vi "Boolean click counter program.vi"() -> ()   [LabVIEW 2021]
panel:
  out "Counts OFF":bool
  out "Turned off":dbl
  in  "Stop While":bool
  out "Turned on":dbl
  in  "Counts ON":bool
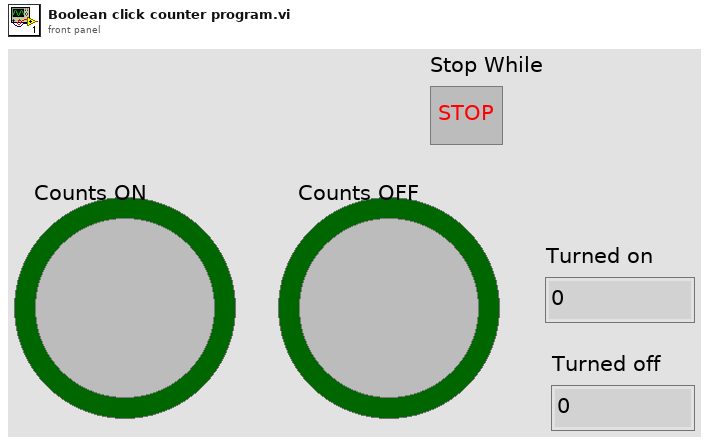
[diagram p1: front panel]
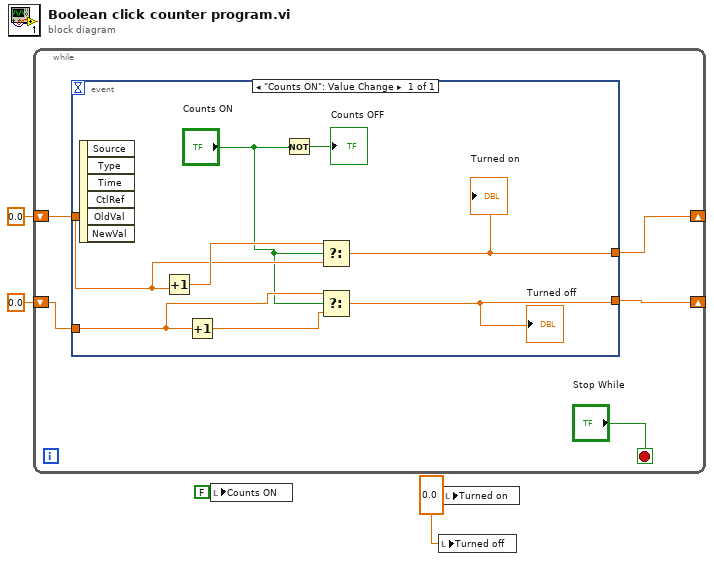
[diagram p0: block diagram]
diagram:
  w3 = 0.0 ("Numeric")
  n1 = while {
    shift-right: [w8] -> _
    shift-left: 0.0 -> [w9]
    shift-right: [w5] -> _
    shift-left: 0.0 -> [w6]
    stop <- "Stop While" stop-if-true
    n2 = event shown="[0] \"Counts ON\": Value Change" {
      selector: _ -> [_]
      dyn-events: _ -> [_]
      timeout: _ -> [_]
      tunnel: w9 -> [w15]
      tunnel: [w16] -> w8
      tunnel: w6 -> [w13]
      tunnel: [w12] -> w5
      event "Counts ON": Value Change {
        n3 = event-data() -> ()  [unwired: 1 in, 6 out]
        n4 = Increment(x=w15) -> (x+1=w17:dbl)
        n5 = Increment(x=w13) -> (x+1=w14:dbl)
        n6 = Not(x="Counts ON") -> (.not. x?=→"Counts OFF":bool)
        n7 = Select(t=w17, s="Counts ON", f=w15) -> (s? t:f=w16:dbl)
        "Turned on" <- w16
        n8 = Select(t=w13, s="Counts ON", f=w14) -> (s? t:f=w12:dbl)
        "Turned off" <- w12
      }
    }
  }
  n9 = local write "Counts ON"(FALSE ("Boolean")) -> ()
  n10 = local write "Turned off"(w3) -> ()
  n11 = local write "Turned on"(w3) -> ()
